vi "main.vi"() -> ()   [LabVIEW 2024]
uses:
  StateVariable.ctl
panel:
  out "Waveform Chart":T1(graph)
  out "State name":string
  in  "Pause":bool
  in  "Start":bool
  in  "Stop":bool
  # "Template : LabVIEW  Event State Machine"
  # "LINE: THAITECHZONE"
  # "State EVENT"
  # "Signal Acquired"
  # "NATTAPHOL JASUNGNUEN"
  # "LINE : @thaitechzone"
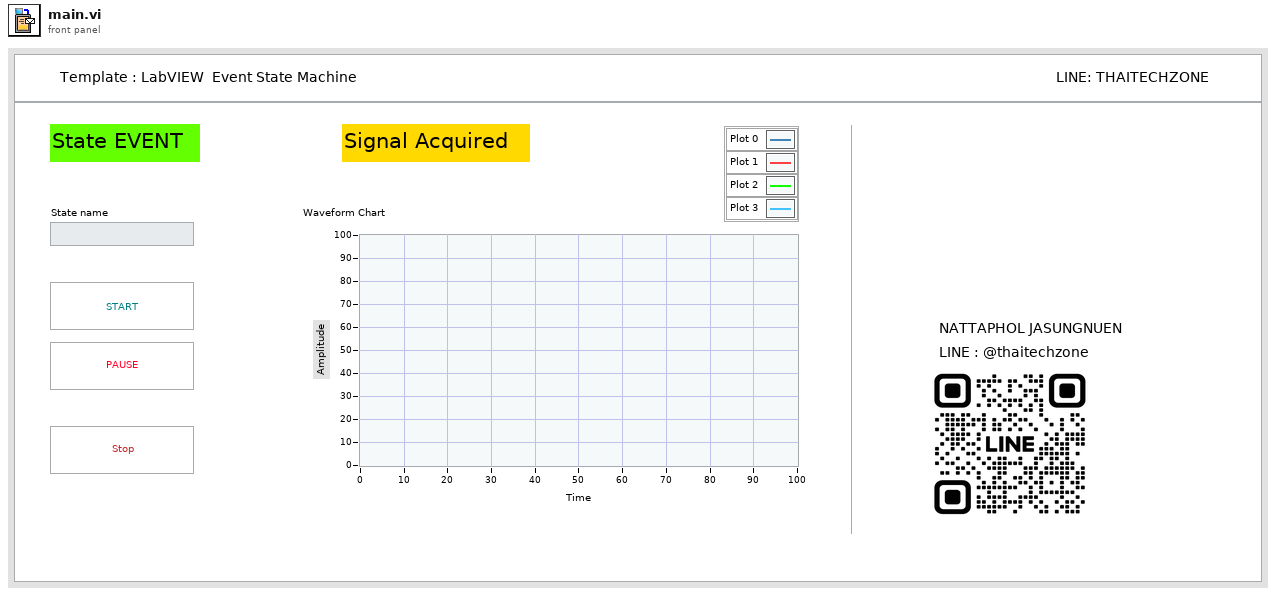
[diagram p1: front panel]
types:
  T1 = cluster{"Array Out[0]":u64, "Array Out[1]":u64, "Array Out[2]":u64, "Array Out[3]":u64, "Array Out[4]":u64, "Array Out[5]":u64, "Array Out[6]":u64, "Array Out[7]":u64, "Array Out[8]":u64}
  T2 = typedef "StateVariable.ctl" = enum16{"Initialization", "Start", "Acquired Data", "Processing", "Update  Display Data", "Logging", "Pause", "WaitForEvent", "Exit"}
  T3 = enum8{"Enabled", "Disabled", "Disabled and Grayed Out"}
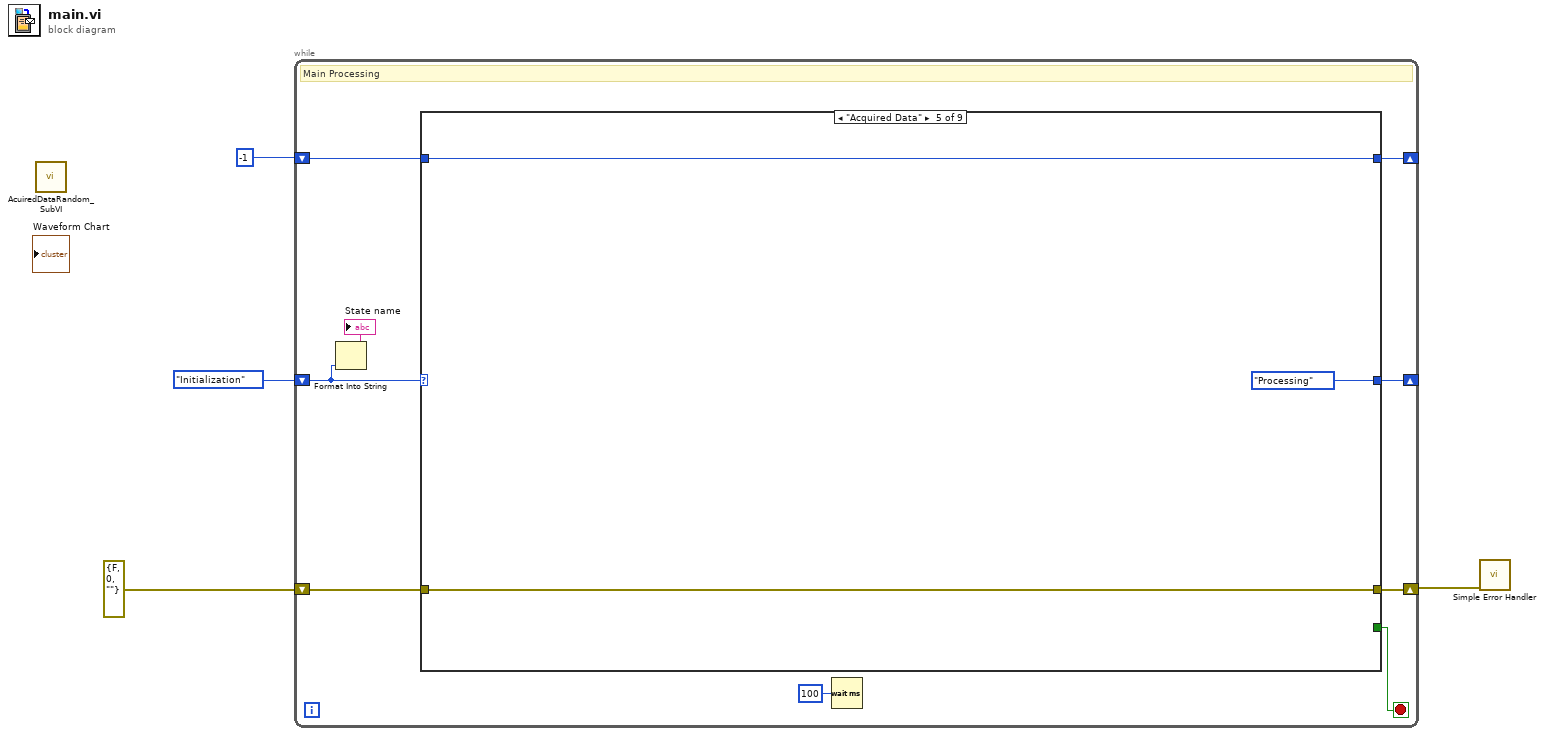
[diagram p0: block diagram]
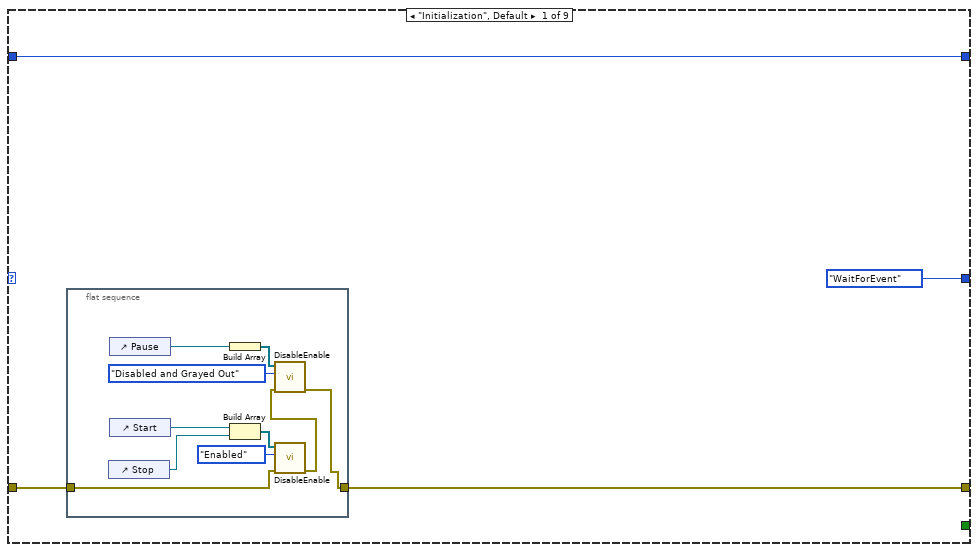
[diagram p2: hidden frame]
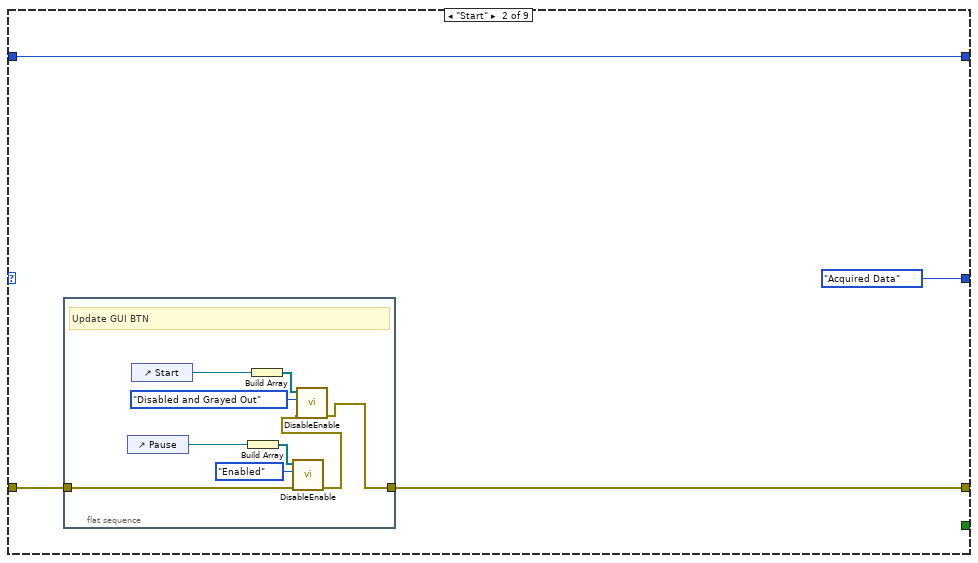
[diagram p3: hidden frame]
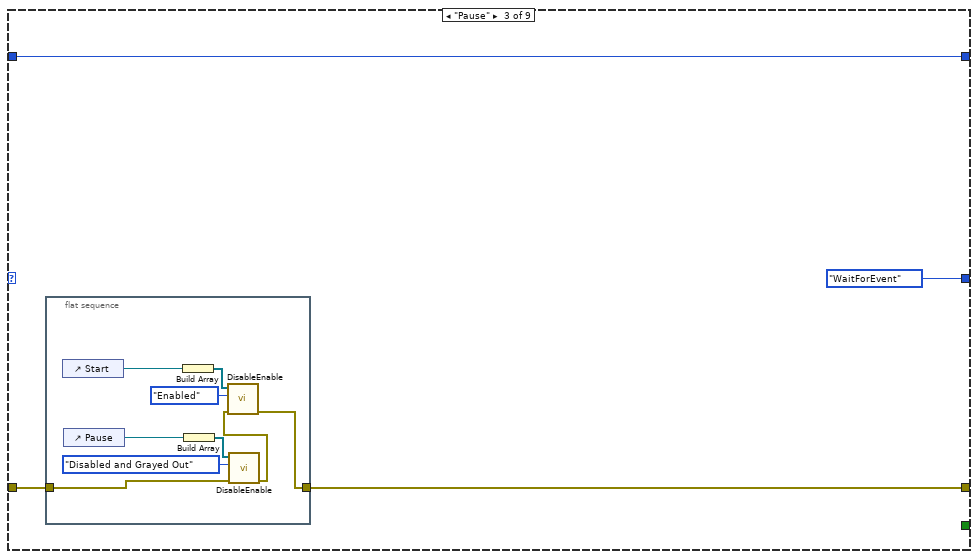
[diagram p4: hidden frame]
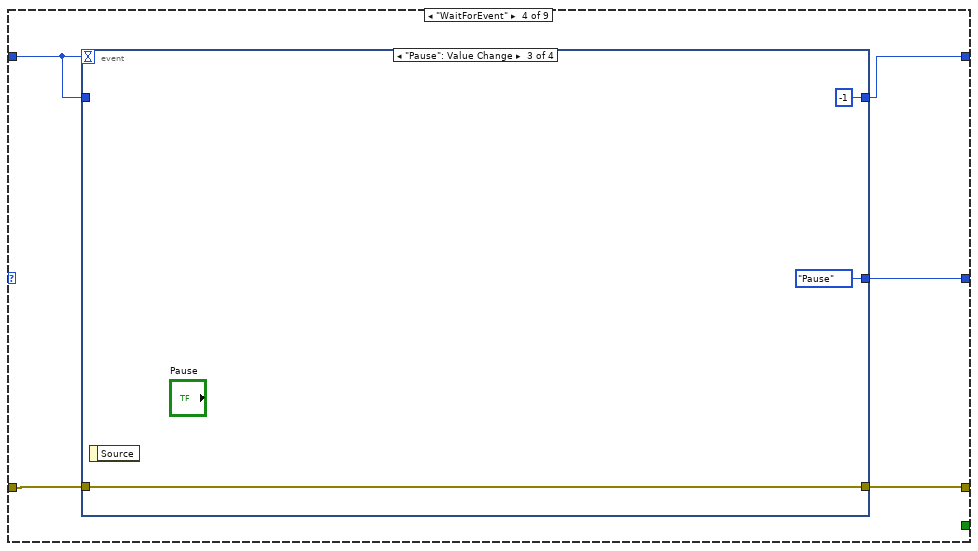
[diagram p5: hidden frame]
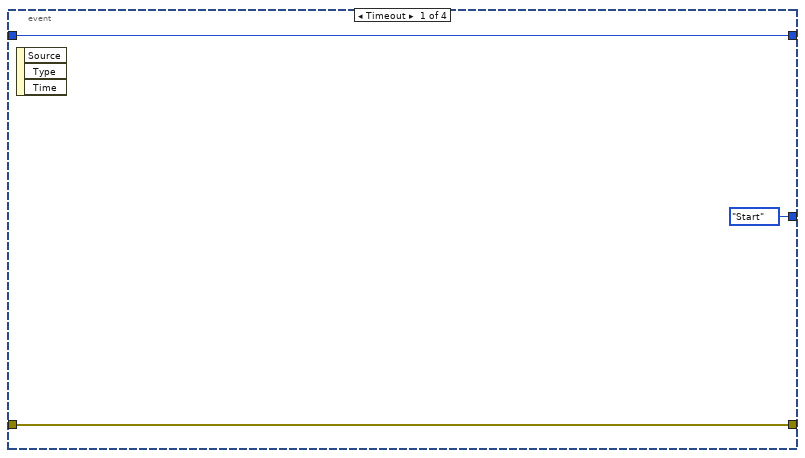
[diagram p6: hidden frame]
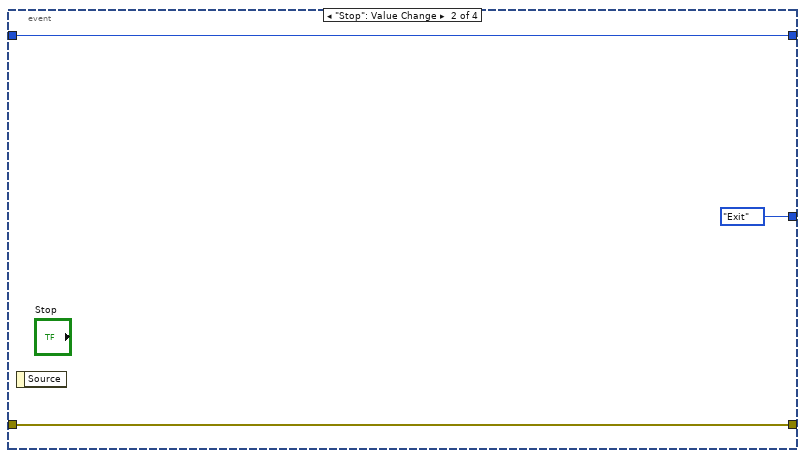
[diagram p7: hidden frame]
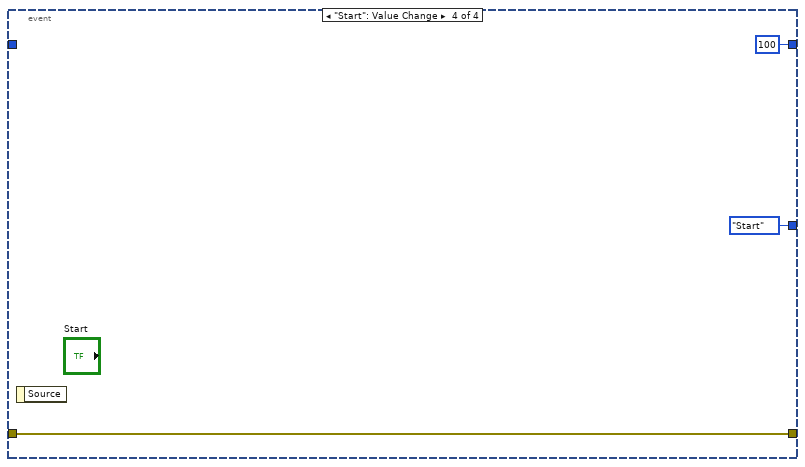
[diagram p8: hidden frame]
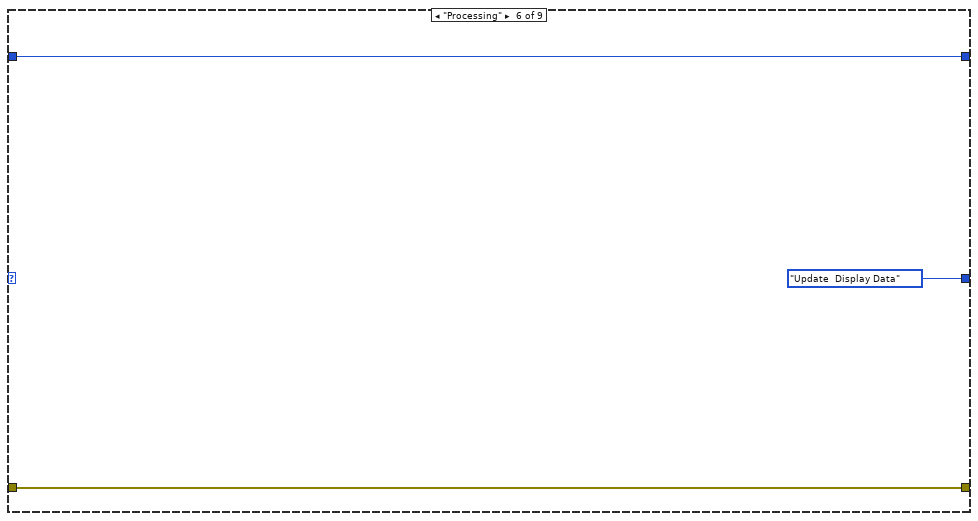
[diagram p9: hidden frame]
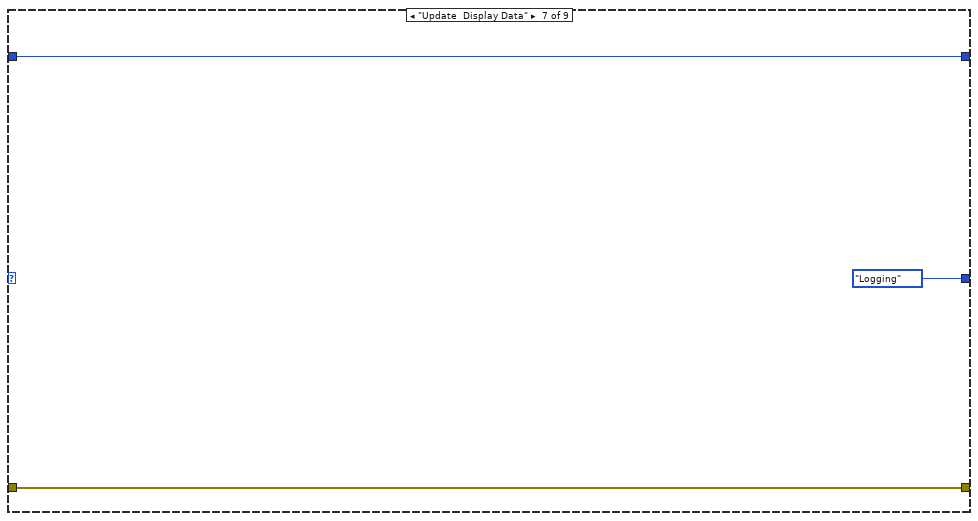
[diagram p10: hidden frame]
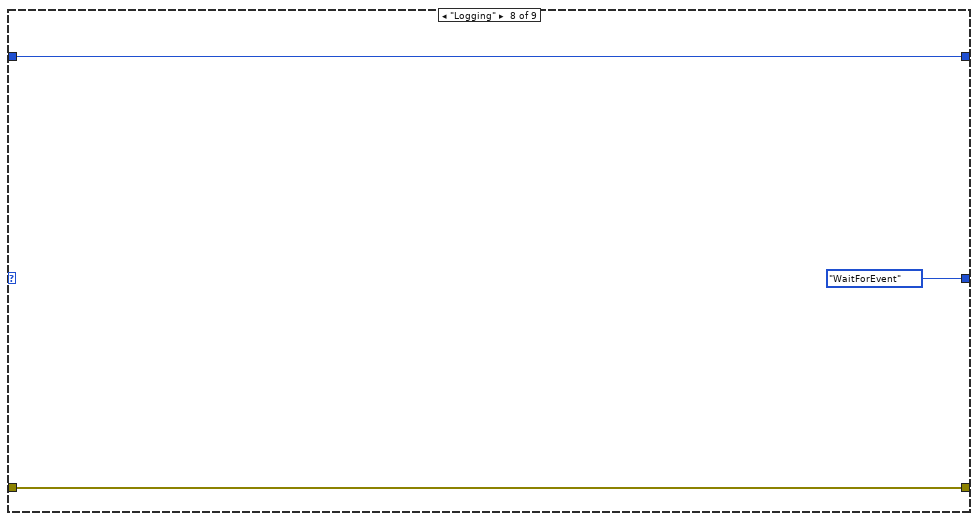
[diagram p11: hidden frame]
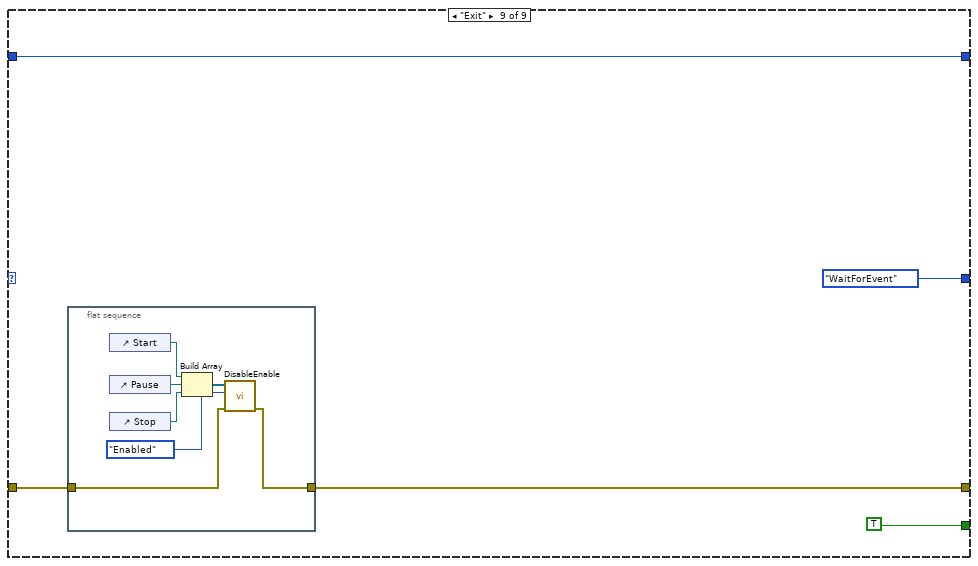
[diagram p12: hidden frame]
diagram:
  n1 = call "AcuiredDataRandom_SubVI.vi"() -> ()  [unwired: 11 in, 1 out]
  n2 = while {
    shift-right: [w13] -> _
    shift-left: StateVariable."Initialization" ("Enum") -> [w12]
    shift-right: [w7] -> _
    shift-left: -1 -> [w8]
    shift-right: [w5] -> w2
    shift-left: errorcluster {"status"=FALSE, "code"=0, "source"=""} ("error constant") -> [w6]
    stop <- w10 stop-if-true
    # "Main Processing"
    n3 = Format Into String(w12) -> (resulting string=→"State name":string)  [unwired: 3 in, 1 out]
    n4 = case shown="\"Acquired Data\"" w12 {
      tunnel: [StateVariable."WaitForEvent" ("Enum") StateVariable."Acquired Data" ("Enum") StateVariable."WaitForEvent" ("Enum") w58 StateVariable."Processing" ("Enum") StateVariable."Update  Display Data" ("Enum") StateVariable."Logging" ("Enum") StateVariable."WaitForEvent" ("Enum") StateVariable."WaitForEvent" ("Enum")] -> w13
      tunnel: [_ _ _ _ _ _ _ _ TRUE] -> w10
      tunnel: w8 -> [w17 w30 w43 w57 w73 w76 w79 w82 w85]
      tunnel: [w17 w30 w43 w56 w73 w76 w79 w82 w85] -> w7
      tunnel: w6 -> [w15 w29 w42 w54 w72 w75 w77 w80 w84]
      tunnel: [w14 w28 w41 w55 w72 w75 w77 w80 w83] -> w5
      frame "Initialization", Default {
        n5 = flat-sequence {
          tunnel: w15 -> [w20]
          tunnel: [w18] -> w14
          frame #0 {
            n6 = control-ref of="Stop"() -> (w21:refnum<vi>)
            n7 = control-ref of="Pause"() -> (w26:refnum<vi>)
            n8 = control-ref of="Start"() -> (w23:refnum<vi>)
            n9 = Build Array(w26) -> (w25:refnum<vi>[])
            n10 = Build Array(w23, w21) -> (w24:refnum<vi>[])
            n11 = call "DisableEnable.vi"("error in (no error)"=w20, "Action"=T3."Enabled", "Array of Control References"=w24) -> ("error out"=w19:errorcluster)  [unwired: 8 in]
            n12 = call "DisableEnable.vi"("error in (no error)"=w19, "Action"=T3."Disabled and Grayed Out", "Array of Control References"=w25) -> ("error out"=w18:errorcluster)  [unwired: 8 in]
          }
        }
      }
      frame "Start" {
        n13 = flat-sequence {
          tunnel: w29 -> [w34]
          tunnel: [w32] -> w28
          frame #0 {
            # "Update GUI BTN"
            n14 = control-ref of="Pause"() -> (w40:refnum<vi>)
            n15 = control-ref of="Start"() -> (w37:refnum<vi>)
            n16 = Build Array(w40) -> (w39:refnum<vi>[])
            n17 = Build Array(w37) -> (w38:refnum<vi>[])
            n18 = call "DisableEnable.vi"("error in (no error)"=w34, "Action"=T3."Enabled", "Array of Control References"=w39) -> ("error out"=w33:errorcluster)  [unwired: 8 in]
            n19 = call "DisableEnable.vi"("error in (no error)"=w33, "Action"=T3."Disabled and Grayed Out", "Array of Control References"=w38) -> ("error out"=w32:errorcluster)  [unwired: 8 in]
          }
        }
      }
      frame "Pause" {
        n20 = flat-sequence {
          tunnel: w42 -> [w46]
          tunnel: [w45] -> w41
          frame #0 {
            n21 = control-ref of="Start"() -> (w53:refnum<vi>)
            n22 = control-ref of="Pause"() -> (w50:refnum<vi>)
            n23 = Build Array(w53) -> (w52:refnum<vi>[])
            n24 = Build Array(w50) -> (w51:refnum<vi>[])
            n25 = call "DisableEnable.vi"("error in (no error)"=w46, "Action"=T3."Disabled and Grayed Out", "Array of Control References"=w51) -> ("error out"=w47:errorcluster)  [unwired: 8 in]
            n26 = call "DisableEnable.vi"("error in (no error)"=w47, "Action"=T3."Enabled", "Array of Control References"=w52) -> ("error out"=w45:errorcluster)  [unwired: 8 in]
          }
        }
      }
      frame "WaitForEvent" {
        n27 = event shown="[2] \"Pause\": Value Change" {
          selector: _ -> [_ _ _ _]
          dyn-events: _ -> [_ _ _ _]
          timeout: w57 -> [_ _ _ _]
          tunnel: [StateVariable."Start" ("Enum") StateVariable."Exit" ("Enum") StateVariable."Pause" ("Enum") StateVariable."Start" ("Enum")] -> w58
          tunnel: [w60 w63 -1 100] -> w56
          tunnel: w57 -> [w60 w63 _ _]
          tunnel: [w59 w62 w65 w68] -> w55
          tunnel: w54 -> [w59 w62 w65 w68]
          event Timeout {
            n28 = event-data() -> ()  [unwired: 1 in, 3 out]
          }
          event "Stop": Value Change {
            n29 = event-data() -> ()  [unwired: 1 in, 1 out]
          }
          event "Pause": Value Change {
            n30 = event-data() -> ()  [unwired: 1 in, 1 out]
          }
          event "Start": Value Change {
            n31 = event-data() -> ()  [unwired: 1 in, 1 out]
          }
        }
      }
      frame "Acquired Data" {
      }
      frame "Processing" {
      }
      frame "Update  Display Data" {
      }
      frame "Logging" {
      }
      frame "Exit" {
        n32 = flat-sequence {
          tunnel: w84 -> [w89]
          tunnel: [w88] -> w83
          frame #0 {
            n33 = control-ref of="Start"() -> (w94:refnum<vi>)
            n34 = control-ref of="Pause"() -> (w92:refnum<vi>)
            n35 = control-ref of="Stop"() -> (w91:refnum<vi>)
            n36 = Build Array(w94, w92, w91) -> (w93:refnum<vi>[])
            n37 = call "DisableEnable.vi"("error in (no error)"=w89, "Action"=T3."Enabled", "Array of Control References"=w93) -> ("error out"=w88:errorcluster)  [unwired: 8 in]
          }
        }
      }
    }
    n38 = Wait (ms)(milliseconds to wait=u32 100) -> ()  [unwired: 1 out]
  }
  n39 = call <vilib>:"Simple Error Handler.vi"("error in (no error)"=w2) -> ()  [unwired: 4 in, 5 out]
